vi "create.vi"(8 "error in":errorcluster, 11 "publish mode":T1) -> (0 "error out":errorcluster, 3 "stream publisher out":refnum<class "data bus stream publisher.lvclass">)   [LabVIEW 2013, in "data bus stream publisher.lvclass"]
uses:
  data bus stream publisher.lvclass
  publish mode.ctl
  data bus stream publisher.lvclass/data bus stream publisher.ctl
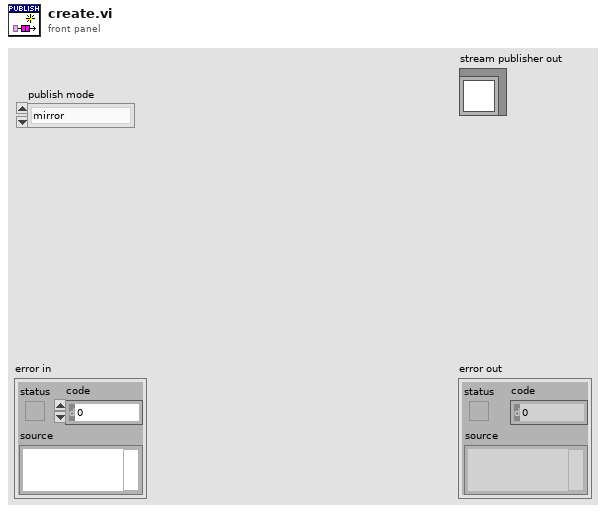
[diagram p1: front panel]
types:
  T1 = typedef "data bus stream publisher.lvclass/publish mode.ctl" = enum16{"mirror", "round robin"}
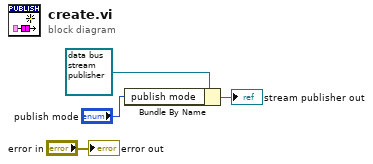
[diagram p0: block diagram]
diagram:
  n1 = Bundle By Name(cluster=refnum<class "data bus stream publisher.lvclass"> refnum ("stream publisher in"), "publish mode"="publish mode") -> (→"stream publisher out":refnum<class "data bus stream publisher.lvclass">)
  "error out" <- "error in"
